vi "Series Recognition.vi"(8 "error in (no error)":errorcluster, 10 "Series Type (0: MXG)":u16(ring) items=["MXG-A", "PSG", "PSG-A", "PSG-C", "PSG-D", "MXG-B", "EXG"], 11 "VISA resource name":refnum<visa-resource-name>) -> (0 "error out":errorcluster, 2 "Is Series Correct":bool, 3 "VISA resource name out":refnum<visa-resource-name>)   [LabVIEW 2018, in "Agilent PSG MXG Series.lvlib"]
doc: "Specifies whether the series is correct."
uses:
  Agilent PSG MXG Series.lvlib
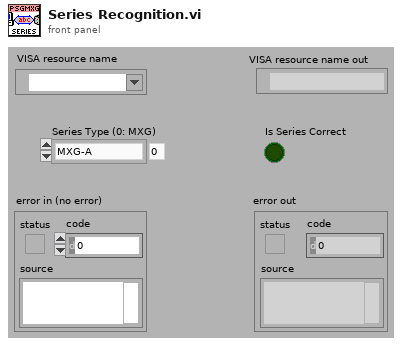
[diagram p1: front panel]
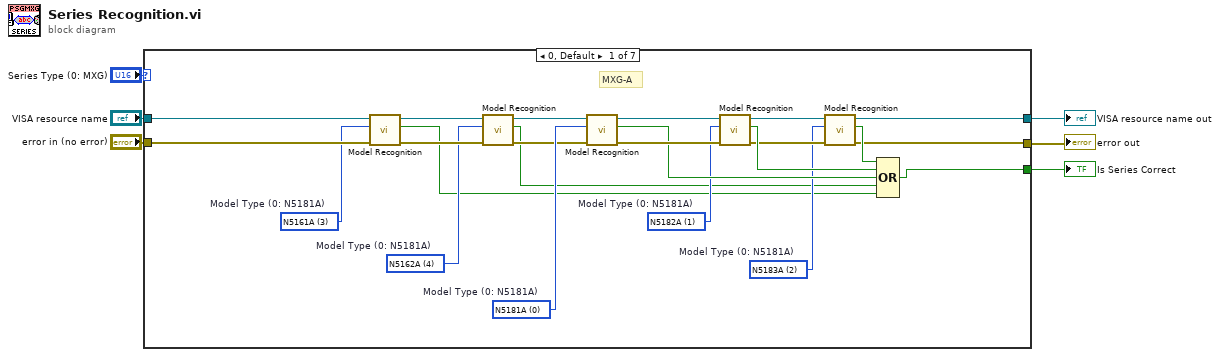
[diagram p0: block diagram]
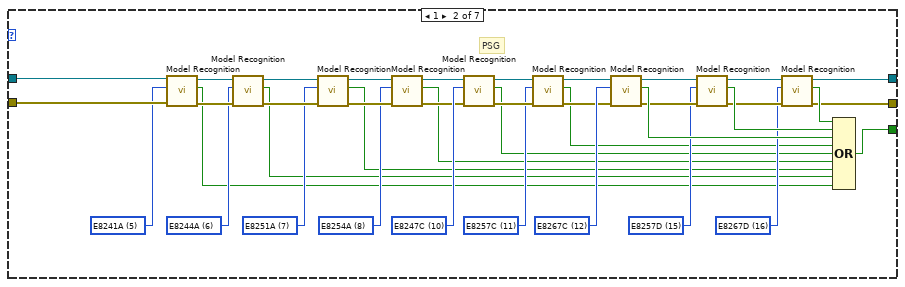
[diagram p2: hidden frame]
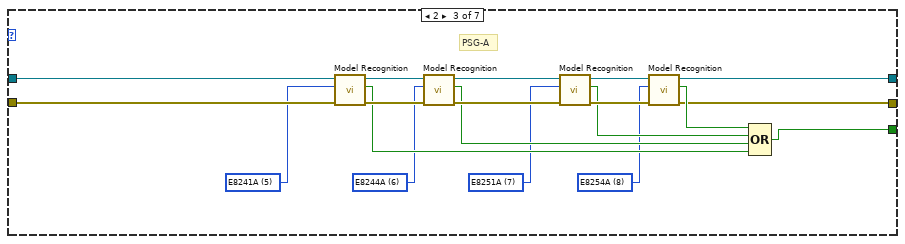
[diagram p3: hidden frame]
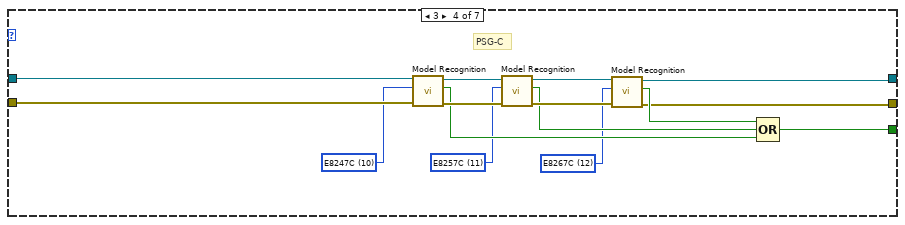
[diagram p4: hidden frame]
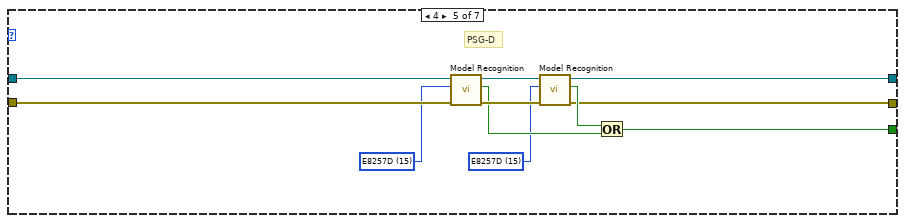
[diagram p5: hidden frame]
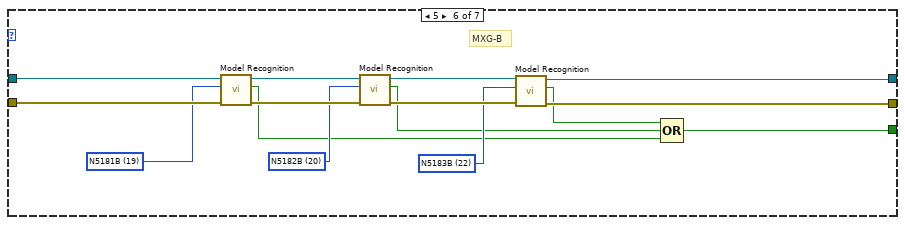
[diagram p6: hidden frame]
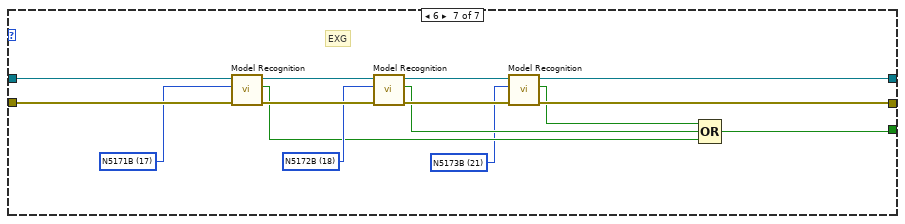
[diagram p7: hidden frame]
diagram:
  n1 = case shown="0, Default" "Series Type (0: MXG)" {
    tunnel: "VISA resource name" -> [w16 w57 w85 w100 w109 w128 w143]
    tunnel: "error in (no error)" -> [w13 w50 w84 w94 w108 w127 w142]
    tunnel: [w21 w62 w75 w93 w107 w120 w136] -> w3
    tunnel: [w8 w30 w69 w88 w104 w119 w134] -> w2
    tunnel: [w7 w31 w70 w89 w103 w114 w129] -> w1
    frame 0, Default {
      w11 = u16 3 items=["N5181A"=0, "N5182A"=1, "N5183A"=2, "N5161A"=3, "N5162A"=4, "E8241A"=5, "E8244A"=6, "E8251A"=7, "E8254A"=8, "E8247C"=10, "E8257C"=11, "E8267C"=12, "E8257D"=15, "E8267D"=16, "N5171B"=17, "N5172B"=18, "N5181B"=19, "N5182B"=20]  # Model Type (0: N5181A)
      w12 = u16 4 items=["N5181A"=0, "N5182A"=1, "N5183A"=2, "N5161A"=3, "N5162A"=4, "E8241A"=5, "E8244A"=6, "E8251A"=7, "E8254A"=8, "E8247C"=10, "E8257C"=11, "E8267C"=12, "E8257D"=15, "E8267D"=16, "N5171B"=17, "N5172B"=18, "N5181B"=19, "N5182B"=20]  # Model Type (0: N5181A)
      w20 = u16 2 items=["N5181A"=0, "N5182A"=1, "N5183A"=2, "E8241A"=5, "E8244A"=6, "E8251A"=7, "E8254A"=8, "E8247C"=10, "E8257C"=11, "E8267C"=12, "E8257D"=15, "E8267D"=16]  # Model Type (0: N5181A)
      w24 = u16 1 items=["N5181A"=0, "N5182A"=1, "E8241A"=5, "E8244A"=6, "E8251A"=7, "E8254A"=8, "E8247C"=10, "E8257C"=11, "E8267C"=12, "E8257D"=15, "E8267D"=16]  # Model Type (0: N5181A)
      w25 = u16 0 items=["N5181A"=0, "N5182A"=1, "E8241A"=5, "E8244A"=6, "E8251A"=7, "E8254A"=8, "E8247C"=10, "E8257C"=11, "E8267C"=12, "E8257D"=15, "E8267D"=16]  # Model Type (0: N5181A)
      # "MXG-A"
      n2 = call "Model Recognition.vi"("error in (no error)"=w13, "Model Type (0: N5181A)"=w11, "VISA resource name"=w16) -> ("error out"=w14:errorcluster, "Is Model Correct"=w9:bool, "VISA resource name out"=w15:refnum<visa-resource-name>)  [unwired: 1 in, 5 out]
      n3 = call "Model Recognition.vi"("error in (no error)"=w14, "Model Type (0: N5181A)"=w12, "VISA resource name"=w15) -> ("error out"=w18:errorcluster, "Is Model Correct"=w10:bool, "VISA resource name out"=w17:refnum<visa-resource-name>)  [unwired: 1 in, 5 out]
      n4 = call "Model Recognition.vi"("error in (no error)"=w18, "Model Type (0: N5181A)"=w25, "VISA resource name"=w17) -> ("error out"=w28:errorcluster, "Is Model Correct"=w27:bool, "VISA resource name out"=w29:refnum<visa-resource-name>)  [unwired: 1 in, 5 out]
      n5 = call "Model Recognition.vi"("error in (no error)"=w28, "Model Type (0: N5181A)"=w24, "VISA resource name"=w29) -> ("error out"=w22:errorcluster, "Is Model Correct"=w26:bool, "VISA resource name out"=w23:refnum<visa-resource-name>)  [unwired: 1 in, 5 out]
      n6 = call "Model Recognition.vi"("error in (no error)"=w22, "Model Type (0: N5181A)"=w20, "VISA resource name"=w23) -> ("error out"=w8:errorcluster, "Is Model Correct"=w19:bool, "VISA resource name out"=w21:refnum<visa-resource-name>)  [unwired: 1 in, 5 out]
      n7 = Compound Arithmetic op=OR(w19, w26, w27, w10, w9) -> (w7:bool)
    }
    frame 1 {
      w39 = u16 5 items=["N5181A"=0, "N5182A"=1, "N5183A"=2, "N5161A"=3, "N5162A"=4, "E8241A"=5, "E8244A"=6, "E8251A"=7, "E8254A"=8, "E8247C"=10, "E8257C"=11, "E8267C"=12, "E8257D"=15, "E8267D"=16, "N5171B"=17, "N5172B"=18, "N5181B"=19, "N5182B"=20] ("Model Type (0: N5181A)")
      w40 = u16 6 items=["N5181A"=0, "N5182A"=1, "N5183A"=2, "N5161A"=3, "N5162A"=4, "E8241A"=5, "E8244A"=6, "E8251A"=7, "E8254A"=8, "E8247C"=10, "E8257C"=11, "E8267C"=12, "E8257D"=15, "E8267D"=16, "N5171B"=17, "N5172B"=18, "N5181B"=19, "N5182B"=20] ("Model Type (0: N5181A)")
      w41 = u16 7 items=["N5181A"=0, "N5182A"=1, "N5183A"=2, "N5161A"=3, "N5162A"=4, "E8241A"=5, "E8244A"=6, "E8251A"=7, "E8254A"=8, "E8247C"=10, "E8257C"=11, "E8267C"=12, "E8257D"=15, "E8267D"=16, "N5171B"=17, "N5172B"=18, "N5181B"=19, "N5182B"=20] ("Model Type (0: N5181A)")
      w42 = u16 8 items=["N5181A"=0, "N5182A"=1, "N5183A"=2, "N5161A"=3, "N5162A"=4, "E8241A"=5, "E8244A"=6, "E8251A"=7, "E8254A"=8, "E8247C"=10, "E8257C"=11, "E8267C"=12, "E8257D"=15, "E8267D"=16, "N5171B"=17, "N5172B"=18, "N5181B"=19, "N5182B"=20] ("Model Type (0: N5181A)")
      w43 = u16 10 items=["N5181A"=0, "N5182A"=1, "N5183A"=2, "N5161A"=3, "N5162A"=4, "E8241A"=5, "E8244A"=6, "E8251A"=7, "E8254A"=8, "E8247C"=10, "E8257C"=11, "E8267C"=12, "E8257D"=15, "E8267D"=16, "N5171B"=17, "N5172B"=18, "N5181B"=19, "N5182B"=20] ("Model Type (0: N5181A)")
      w44 = u16 11 items=["N5181A"=0, "N5182A"=1, "N5183A"=2, "N5161A"=3, "N5162A"=4, "E8241A"=5, "E8244A"=6, "E8251A"=7, "E8254A"=8, "E8247C"=10, "E8257C"=11, "E8267C"=12, "E8257D"=15, "E8267D"=16, "N5171B"=17, "N5172B"=18, "N5181B"=19, "N5182B"=20] ("Model Type (0: N5181A)")
      w58 = u16 12 items=["N5181A"=0, "N5182A"=1, "N5183A"=2, "N5161A"=3, "N5162A"=4, "E8241A"=5, "E8244A"=6, "E8251A"=7, "E8254A"=8, "E8247C"=10, "E8257C"=11, "E8267C"=12, "E8257D"=15, "E8267D"=16, "N5171B"=17, "N5172B"=18, "N5181B"=19, "N5182B"=20] ("Model Type (0: N5181A)")
      w59 = u16 15 items=["N5181A"=0, "N5182A"=1, "N5183A"=2, "N5161A"=3, "N5162A"=4, "E8241A"=5, "E8244A"=6, "E8251A"=7, "E8254A"=8, "E8247C"=10, "E8257C"=11, "E8267C"=12, "E8257D"=15, "E8267D"=16, "N5171B"=17, "N5172B"=18, "N5181B"=19, "N5182B"=20] ("Model Type (0: N5181A)")
      w60 = u16 16 items=["N5181A"=0, "N5182A"=1, "N5183A"=2, "N5161A"=3, "N5162A"=4, "E8241A"=5, "E8244A"=6, "E8251A"=7, "E8254A"=8, "E8247C"=10, "E8257C"=11, "E8267C"=12, "E8257D"=15, "E8267D"=16, "N5171B"=17, "N5172B"=18, "N5181B"=19, "N5182B"=20] ("Model Type (0: N5181A)")
      # "PSG"
      n8 = call "Model Recognition.vi"("error in (no error)"=w50, "Model Type (0: N5181A)"=w39, "VISA resource name"=w57) -> ("error out"=w49:errorcluster, "Is Model Correct"=w32:bool, "VISA resource name out"=w56:refnum<visa-resource-name>)  [unwired: 1 in, 5 out]
      n9 = call "Model Recognition.vi"("error in (no error)"=w49, "Model Type (0: N5181A)"=w40, "VISA resource name"=w56) -> ("error out"=w48:errorcluster, "Is Model Correct"=w33:bool, "VISA resource name out"=w55:refnum<visa-resource-name>)  [unwired: 1 in, 5 out]
      n10 = call "Model Recognition.vi"("error in (no error)"=w48, "Model Type (0: N5181A)"=w41, "VISA resource name"=w55) -> ("error out"=w47:errorcluster, "Is Model Correct"=w34:bool, "VISA resource name out"=w54:refnum<visa-resource-name>)  [unwired: 1 in, 5 out]
      n11 = call "Model Recognition.vi"("error in (no error)"=w47, "Model Type (0: N5181A)"=w42, "VISA resource name"=w54) -> ("error out"=w37:errorcluster, "Is Model Correct"=w35:bool, "VISA resource name out"=w53:refnum<visa-resource-name>)  [unwired: 1 in, 5 out]
      n12 = call "Model Recognition.vi"("error in (no error)"=w37, "Model Type (0: N5181A)"=w43, "VISA resource name"=w53) -> ("error out"=w46:errorcluster, "Is Model Correct"=w36:bool, "VISA resource name out"=w52:refnum<visa-resource-name>)  [unwired: 1 in, 5 out]
      n13 = call "Model Recognition.vi"("error in (no error)"=w46, "Model Type (0: N5181A)"=w44, "VISA resource name"=w52) -> ("error out"=w45:errorcluster, "Is Model Correct"=w38:bool, "VISA resource name out"=w51:refnum<visa-resource-name>)  [unwired: 1 in, 5 out]
      n14 = call "Model Recognition.vi"("error in (no error)"=w45, "Model Type (0: N5181A)"=w58, "VISA resource name"=w51) -> ("error out"=w66:errorcluster, "Is Model Correct"=w67:bool, "VISA resource name out"=w65:refnum<visa-resource-name>)  [unwired: 1 in, 5 out]
      n15 = call "Model Recognition.vi"("error in (no error)"=w66, "Model Type (0: N5181A)"=w59, "VISA resource name"=w65) -> ("error out"=w63:errorcluster, "Is Model Correct"=w68:bool, "VISA resource name out"=w64:refnum<visa-resource-name>)  [unwired: 1 in, 5 out]
      n16 = call "Model Recognition.vi"("error in (no error)"=w63, "Model Type (0: N5181A)"=w60, "VISA resource name"=w64) -> ("error out"=w30:errorcluster, "Is Model Correct"=w61:bool, "VISA resource name out"=w62:refnum<visa-resource-name>)  [unwired: 1 in, 5 out]
      n17 = Compound Arithmetic op=OR(w61, w68, w67, w38, w36, w35, w34, w33, w32) -> (w31:bool)
    }
    frame 2 {
      w71 = u16 8 items=["N5181A"=0, "N5182A"=1, "E8241A"=5, "E8244A"=6, "E8251A"=7, "E8254A"=8, "E8247C"=10, "E8257C"=11, "E8267C"=12, "E8257D"=15, "E8267D"=16] ("Model Type (0: N5181A)")
      w72 = u16 7 items=["N5181A"=0, "N5182A"=1, "E8241A"=5, "E8244A"=6, "E8251A"=7, "E8254A"=8, "E8247C"=10, "E8257C"=11, "E8267C"=12, "E8257D"=15, "E8267D"=16] ("Model Type (0: N5181A)")
      w73 = u16 6 items=["N5181A"=0, "N5182A"=1, "E8241A"=5, "E8244A"=6, "E8251A"=7, "E8254A"=8, "E8247C"=10, "E8257C"=11, "E8267C"=12, "E8257D"=15, "E8267D"=16] ("Model Type (0: N5181A)")
      w74 = u16 5 items=["N5181A"=0, "N5182A"=1, "E8241A"=5, "E8244A"=6, "E8251A"=7, "E8254A"=8, "E8247C"=10, "E8257C"=11, "E8267C"=12, "E8257D"=15, "E8267D"=16] ("Model Type (0: N5181A)")
      # "PSG-A"
      n18 = call "Model Recognition.vi"("error in (no error)"=w84, "Model Type (0: N5181A)"=w74, "VISA resource name"=w85) -> ("error out"=w87:errorcluster, "Is Model Correct"=w79:bool, "VISA resource name out"=w86:refnum<visa-resource-name>)  [unwired: 1 in, 5 out]
      n19 = call "Model Recognition.vi"("error in (no error)"=w87, "Model Type (0: N5181A)"=w73, "VISA resource name"=w86) -> ("error out"=w80:errorcluster, "Is Model Correct"=w78:bool, "VISA resource name out"=w81:refnum<visa-resource-name>)  [unwired: 1 in, 5 out]
      n20 = call "Model Recognition.vi"("error in (no error)"=w80, "Model Type (0: N5181A)"=w72, "VISA resource name"=w81) -> ("error out"=w83:errorcluster, "Is Model Correct"=w77:bool, "VISA resource name out"=w82:refnum<visa-resource-name>)  [unwired: 1 in, 5 out]
      n21 = call "Model Recognition.vi"("error in (no error)"=w83, "Model Type (0: N5181A)"=w71, "VISA resource name"=w82) -> ("error out"=w69:errorcluster, "Is Model Correct"=w76:bool, "VISA resource name out"=w75:refnum<visa-resource-name>)  [unwired: 1 in, 5 out]
      n22 = Compound Arithmetic op=OR(w76, w77, w78, w79) -> (w70:bool)
    }
    frame 3 {
      w90 = u16 12 items=["N5181A"=0, "N5182A"=1, "E8241A"=5, "E8244A"=6, "E8251A"=7, "E8254A"=8, "E8247C"=10, "E8257C"=11, "E8267C"=12, "E8257D"=15, "E8267D"=16] ("Model Type (0: N5181A)")
      w91 = u16 11 items=["N5181A"=0, "N5182A"=1, "E8241A"=5, "E8244A"=6, "E8251A"=7, "E8254A"=8, "E8247C"=10, "E8257C"=11, "E8267C"=12, "E8257D"=15, "E8267D"=16] ("Model Type (0: N5181A)")
      w92 = u16 10 items=["N5181A"=0, "N5182A"=1, "E8241A"=5, "E8244A"=6, "E8251A"=7, "E8254A"=8, "E8247C"=10, "E8257C"=11, "E8267C"=12, "E8257D"=15, "E8267D"=16] ("Model Type (0: N5181A)")
      # "PSG-C"
      n23 = call "Model Recognition.vi"("error in (no error)"=w94, "Model Type (0: N5181A)"=w92, "VISA resource name"=w100) -> ("error out"=w102:errorcluster, "Is Model Correct"=w97:bool, "VISA resource name out"=w101:refnum<visa-resource-name>)  [unwired: 1 in, 5 out]
      n24 = call "Model Recognition.vi"("error in (no error)"=w102, "Model Type (0: N5181A)"=w91, "VISA resource name"=w101) -> ("error out"=w98:errorcluster, "Is Model Correct"=w96:bool, "VISA resource name out"=w99:refnum<visa-resource-name>)  [unwired: 1 in, 5 out]
      n25 = call "Model Recognition.vi"("error in (no error)"=w98, "Model Type (0: N5181A)"=w90, "VISA resource name"=w99) -> ("error out"=w88:errorcluster, "Is Model Correct"=w95:bool, "VISA resource name out"=w93:refnum<visa-resource-name>)  [unwired: 1 in, 5 out]
      n26 = Compound Arithmetic op=OR(w95, w96, w97) -> (w89:bool)
    }
    frame 4 {
      w105 = u16 15 items=["N5181A"=0, "N5182A"=1, "E8241A"=5, "E8244A"=6, "E8251A"=7, "E8254A"=8, "E8247C"=10, "E8257C"=11, "E8267C"=12, "E8257D"=15, "E8267D"=16] ("Model Type (0: N5181A)")
      w106 = u16 15 items=["N5181A"=0, "N5182A"=1, "E8241A"=5, "E8244A"=6, "E8251A"=7, "E8254A"=8, "E8247C"=10, "E8257C"=11, "E8267C"=12, "E8257D"=15, "E8267D"=16] ("Model Type (0: N5181A)")
      # "PSG-D"
      n27 = call "Model Recognition.vi"("error in (no error)"=w108, "Model Type (0: N5181A)"=w106, "VISA resource name"=w109) -> ("error out"=w112:errorcluster, "Is Model Correct"=w111:bool, "VISA resource name out"=w113:refnum<visa-resource-name>)  [unwired: 1 in, 5 out]
      n28 = call "Model Recognition.vi"("error in (no error)"=w112, "Model Type (0: N5181A)"=w105, "VISA resource name"=w113) -> ("error out"=w104:errorcluster, "Is Model Correct"=w110:bool, "VISA resource name out"=w107:refnum<visa-resource-name>)  [unwired: 1 in, 5 out]
      n29 = Or(x=w110, y=w111) -> (x .or. y?=w103:bool)
    }
    frame 5 {
      w118 = u16 22 items=["N5181A"=0, "N5182A"=1, "N5183A"=2, "N5161A"=3, "N5162A"=4, "E8241A"=5, "E8244A"=6, "E8251A"=7, "E8254A"=8, "E8247C"=10, "E8257C"=11, "E8267C"=12, "E8257D"=15, "E8267D"=16, "N5171B"=17, "N5172B"=18, "N5181B"=19, "N5182B"=20, "N5173B"=21, "N5183B"=22] ("Model Type (0: N5181A)")
      w123 = u16 19 items=["N5181A"=0, "N5182A"=1, "N5183A"=2, "N5161A"=3, "N5162A"=4, "E8241A"=5, "E8244A"=6, "E8251A"=7, "E8254A"=8, "E8247C"=10, "E8257C"=11, "E8267C"=12, "E8257D"=15, "E8267D"=16, "N5171B"=17, "N5172B"=18, "N5181B"=19, "N5182B"=20] ("Model Type (0: N5181A)")
      w124 = u16 20 items=["N5181A"=0, "N5182A"=1, "N5183A"=2, "N5161A"=3, "N5162A"=4, "E8241A"=5, "E8244A"=6, "E8251A"=7, "E8254A"=8, "E8247C"=10, "E8257C"=11, "E8267C"=12, "E8257D"=15, "E8267D"=16, "N5171B"=17, "N5172B"=18, "N5181B"=19, "N5182B"=20] ("Model Type (0: N5181A)")
      # "MXG-B"
      n30 = call "Model Recognition.vi"("error in (no error)"=w127, "Model Type (0: N5181A)"=w123, "VISA resource name"=w128) -> ("error out"=w125:errorcluster, "Is Model Correct"=w117:bool, "VISA resource name out"=w126:refnum<visa-resource-name>)  [unwired: 1 in, 5 out]
      n31 = call "Model Recognition.vi"("error in (no error)"=w125, "Model Type (0: N5181A)"=w124, "VISA resource name"=w126) -> ("error out"=w122:errorcluster, "Is Model Correct"=w116:bool, "VISA resource name out"=w121:refnum<visa-resource-name>)  [unwired: 1 in, 5 out]
      n32 = call "Model Recognition.vi"("error in (no error)"=w122, "Model Type (0: N5181A)"=w118, "VISA resource name"=w121) -> ("error out"=w119:errorcluster, "Is Model Correct"=w115:bool, "VISA resource name out"=w120:refnum<visa-resource-name>)  [unwired: 1 in, 5 out]
      n33 = Compound Arithmetic op=OR(w115, w116, w117) -> (w114:bool)
    }
    frame 6 {
      w130 = u16 21 items=["N5181A"=0, "N5182A"=1, "N5183A"=2, "N5161A"=3, "N5162A"=4, "E8241A"=5, "E8244A"=6, "E8251A"=7, "E8254A"=8, "E8247C"=10, "E8257C"=11, "E8267C"=12, "E8257D"=15, "E8267D"=16, "N5171B"=17, "N5172B"=18, "N5181B"=19, "N5182B"=20, "N5173B"=21, "N5183B"=22] ("Model Type (0: N5181A)")
      w138 = u16 17 items=["N5181A"=0, "N5182A"=1, "N5183A"=2, "N5161A"=3, "N5162A"=4, "E8241A"=5, "E8244A"=6, "E8251A"=7, "E8254A"=8, "E8247C"=10, "E8257C"=11, "E8267C"=12, "E8257D"=15, "E8267D"=16, "N5171B"=17, "N5172B"=18, "N5181B"=19, "N5182B"=20] ("Model Type (0: N5181A)")
      w139 = u16 18 items=["N5181A"=0, "N5182A"=1, "N5183A"=2, "N5161A"=3, "N5162A"=4, "E8241A"=5, "E8244A"=6, "E8251A"=7, "E8254A"=8, "E8247C"=10, "E8257C"=11, "E8267C"=12, "E8257D"=15, "E8267D"=16, "N5171B"=17, "N5172B"=18, "N5181B"=19, "N5182B"=20] ("Model Type (0: N5181A)")
      # "EXG"
      n34 = call "Model Recognition.vi"("error in (no error)"=w142, "Model Type (0: N5181A)"=w138, "VISA resource name"=w143) -> ("error out"=w140:errorcluster, "Is Model Correct"=w131:bool, "VISA resource name out"=w141:refnum<visa-resource-name>)  [unwired: 1 in, 5 out]
      n35 = call "Model Recognition.vi"("error in (no error)"=w140, "Model Type (0: N5181A)"=w139, "VISA resource name"=w141) -> ("error out"=w135:errorcluster, "Is Model Correct"=w132:bool, "VISA resource name out"=w137:refnum<visa-resource-name>)  [unwired: 1 in, 5 out]
      n36 = call "Model Recognition.vi"("error in (no error)"=w135, "Model Type (0: N5181A)"=w130, "VISA resource name"=w137) -> ("error out"=w134:errorcluster, "Is Model Correct"=w133:bool, "VISA resource name out"=w136:refnum<visa-resource-name>)  [unwired: 1 in, 5 out]
      n37 = Compound Arithmetic op=OR(w133, w132, w131) -> (w129:bool)
    }
  }
  "error out" <- w2
  "VISA resource name out" <- w3
  "Is Series Correct" <- w1
